vi "cRIO_4DoF_Encoders_countsvel2radvel(subVI).vi"() -> (3 "Joint_space_velocity":dbl[](array[numeric]))   [LabVIEW 2019]
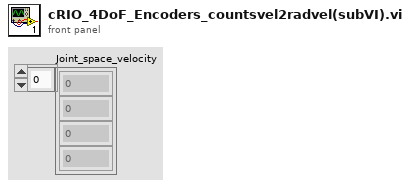
[diagram p1: front panel]
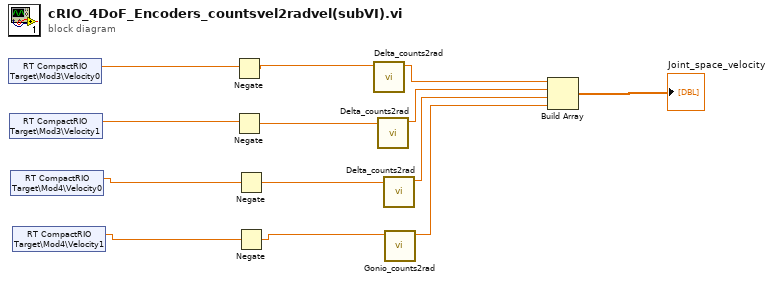
[diagram p0: block diagram]
diagram:
  n1 = shared-variable "RT CompactRIO Target\\Mod3\\Velocity0"() -> (w5:dbl)  [unwired: 1 in, 1 out]
  n2 = shared-variable "RT CompactRIO Target\\Mod3\\Velocity1"() -> (w6:dbl)  [unwired: 1 in, 1 out]
  n3 = shared-variable "RT CompactRIO Target\\Mod4\\Velocity0"() -> (w7:dbl)  [unwired: 1 in, 1 out]
  n4 = shared-variable "RT CompactRIO Target\\Mod4\\Velocity1"() -> (w8:dbl)  [unwired: 1 in, 1 out]
  n5 = Negate(x=w5) -> (-x=w4:dbl)
  n6 = Negate(x=w6) -> (-x=w3:dbl)
  n7 = Negate(x=w7) -> (-x=w2:dbl)
  n8 = Negate(x=w8) -> (-x=w1:dbl)
  n9 = call "Delta_counts2rad.vi"("Numeric in"=w4) -> ("Numeric"=w9:dbl)  [unwired: 10 in]
  n10 = call "Delta_counts2rad.vi"("Numeric in"=w3) -> ("Numeric"=w10:dbl)  [unwired: 10 in]
  n11 = call "Delta_counts2rad.vi"("Numeric in"=w2) -> ("Numeric"=w11:dbl)  [unwired: 10 in]
  n12 = call "Gonio_counts2rad.vi"("Numeric in"=w1) -> ("Numeric"=w12:dbl)  [unwired: 10 in]
  n13 = Build Array(w9, w10, w11, w12) -> (→"Joint_space_velocity":dbl[])
